vi "ExReadPMIFile.vi"() -> ()   [LabVIEW 2010]
panel:
  in  "Full File Name":path
  in  "?":bool
  out "error out":errorcluster
  in  "error in (no error)":errorcluster
  # "NOTICE\n\nTHIS VI REQUIRES THAT THE TOOLKIT\nBE UNLOADED BY RUNNING THE\n VI EXCLOSEGLOBALCAM.VI\n BEFORE LEAVING LABVIEW."
  # "ExReadPMIFile.vi\nThis VI will read a PMI type image file and\ndisplay it.  Be sure to hit the CLOSE IMAGE\nbutton when finished viewing the image so\nit is closed and memory is deallocated\nproperly"
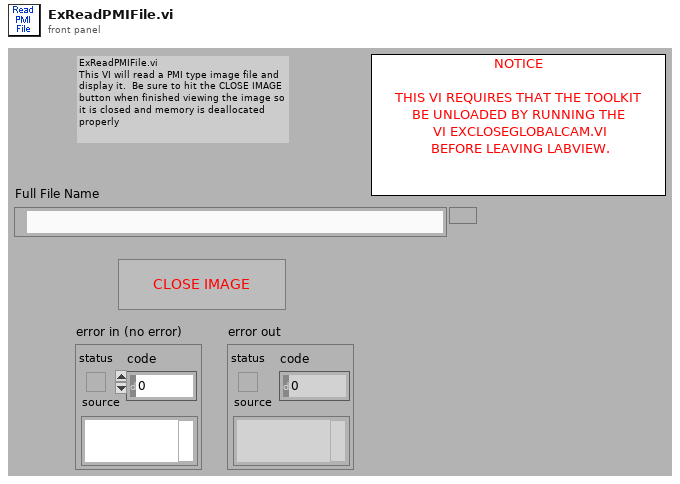
[diagram p1: front panel]
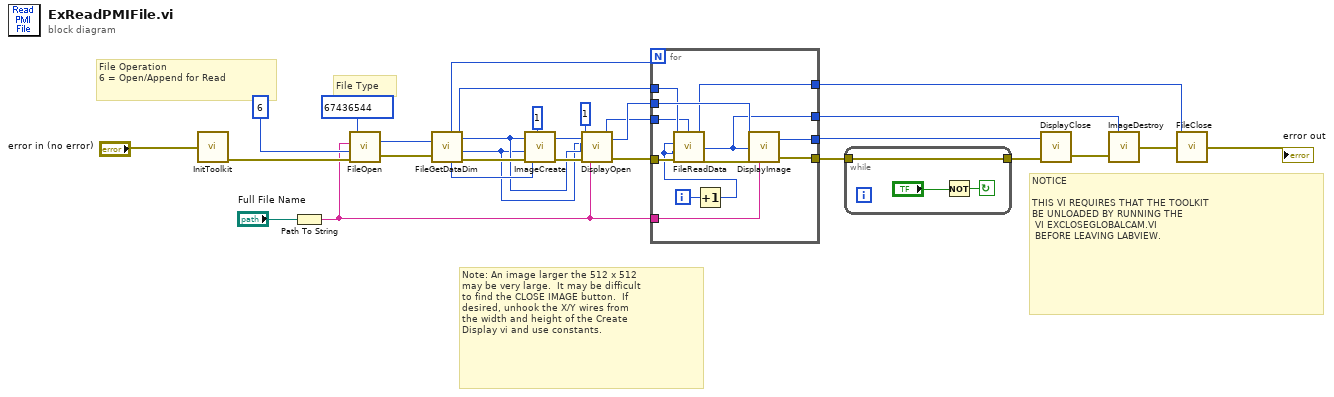
[diagram p0: block diagram]
diagram:
  # "NOTICE\n\nTHIS VI REQUIRES THAT THE TOOLKIT\nBE UNLOADED BY RUNNING THE\n VI EXCLOSEGLOBALCAM.VI\n BEFORE LEAVING LABVIEW."
  # "File Type"
  # "File Operation\n6 = Open/Append for Read"
  # "Note: An image larger the 512 x 512\nmay be very large.  It may be difficult\nto find the CLOSE IMAGE button.  If\ndesired, unhook the X/Y wires from\nthe width and height of the Create\nDisplay vi and use constants."
  n1 = call <userlib>:"InitToolkit.vi"("error in"="error in (no error)") -> ("error out"=w26:errorcluster)
  n2 = Path To String(path="Full File Name") -> (string=w4:string)
  n3 = call <userlib>:"FileOpen.vi"("error in"=w26, "File Operations"=u32 6 ("File Operation"), "FileName"=w4, "File Type"=u32 67436544 ("FileType")) -> ("error out"=w24:errorcluster, "File Handle"=w23:u32)
  n4 = call <userlib>:"FileGetDataDim.vi"("File Handle"=w23, "error in"=w24) -> ("Number of Frames"=w19:u32, "Data Type"=w21:u32, "File Handle"=w14:u32, "X dim"=w3:u32, "Y dim"=w2:u32, "error out"=w22:errorcluster)
  n5 = call <userlib>:"ImageCreate.vi"("X dimension"=w3, "Y dimension"=w2, "Data Type"=w21, "error in"=w22, "Number Of Frames"=1) -> ("Image Handle"=w13:u32, "error out"=w20:errorcluster)
  n6 = call <userlib>:"DisplayOpen.vi"("Display Title"=w4, "Image Handle"=w13, "error in"=w20, "Display Height"=w2, "Display Width"=w3, "Display Type"=1) -> ("error out"=w16:errorcluster, "Display Handle"=w15:u32)
  n7 = for {
    N: w19 -> [_]
    tunnel: w16 -> [w40]
    tunnel: w15 -> [w38]
    tunnel: w14 -> [w37]
    tunnel: w13 -> [w36]
    tunnel: [w33] -> w6
    tunnel: [w32] -> w12
    tunnel: [w31] -> w11
    tunnel: [w30] -> w8
    tunnel: w4 -> [w29]
    i -> [w35]
    n8 = Increment(x=w35) -> (x+1=w34:i32)
    n9 = call <userlib>:"FileReadData.vi"("File Handle"=w37, "Start Frame"=w34, "End Frame"=w34, "error in"=w40, "Image Handle"=w36) -> ("File Handle"=w31:u32, "Image Handle"=w30:u32, "error out"=w39:errorcluster)
    n10 = call <userlib>:"DisplayImage.vi"("error in"=w39, "Title"=w29, "Image Handle"=w30, "Display Handle"=w38) -> ("error out"=w33:errorcluster, "Display Handle"=w32:u32)
  }
  n11 = while {
    tunnel: w6 -> [w43]
    tunnel: [w43] -> w7
    stop <- w41 continue-if-true
    n12 = Not(x="?") -> (.not. x?=w41:bool)
  }
  n13 = call <userlib>:"DisplayClose.vi"("error in"=w7, "Display Handle"=w12) -> ("error out"=w10:errorcluster)
  n14 = call <userlib>:"ImageDestroy.vi"("error in"=w10, "Data handle"=w8) -> ("error out"=w9:errorcluster)
  n15 = call <userlib>:"FileClose.vi"("error in"=w9, "File Handle"=w11) -> ("error out"=→"error out":errorcluster)
